vi "Main.vi"() -> ()   [LabVIEW 2021, in "Main.lvlib"]
uses:
  Main.lvlib
  Init/ReadInitCFG/TypeDef/CFG_Cluster.ctl
  TimeBasedProd/TimeTable/TypeDef/Time_Table.ctl
  TimeBasedProd/TimeTable/TypeDef/Time_Table_CTR.ctl
  TimeBasedProd/Digital_OP/TypeDef/Plant_OP_Map.ctl
  TimeBasedProd/Digital_OP/TypeDef/Plant_OP_Map_CTR.ctl
  ValveCTRL/TypeDef/CHs_List.ctl
  ValveCTRL/TypeDef/ChannelStatus.ctl
  ValveCTRL/TypeDef/Read_Write.ctl
  TimeBasedProd/TypeDef/Read_Write.ctl
  TimeBasedProd/TypeDef/TimeOutInfo.ctl
  ValveCTRL/TypeDef/Queue_Cluster.ctl
  ValveCTRL/TypeDef/States_Enum.ctl
  TimeBasedProd/TypeDef/UpdateTimeOutinfo.ctl
  Init/ReadInitCFG/TypeDef/Operation.ctl
  TimeBasedProd/TimeBasedProd.lvlib
  ValveCTRL/ValveCTRL.lvlib
  Temp_AS6200/Temp_AS6200.lvlib
panel:
  out "CHSt":T1
  in  "Plants_Digital_OP":T2 {"Channel No" items=["7"=7, "11"=11, "12"=12, "13"=13, "15"=15, "16"=16, "18"=18, "29"=29, "32"=32, "33"=33, "35"=35, "36"=36, "37"=37, "38"=38, "40"=40]}
  in  "Time Table":T5 {"Liter" min=0.0; "Set Time" format="%<%H:%M:%S>t"; "Duration[S]" min=0.0}
  in  "cmd":string
  in  "SendCMD":bool
  in  "CFG":T7 {"SystemResetTime" format="%<%H:%M:%S>t"}
  # "Valve -Open Valve -38 -10\nValve -Open Pump -38 -10\nValve -Wait Valve -38 -10\nValve -Close Pump -38 -10\nValve -Close Valve -38 -10"
  # "Event -[Init_IOs,ReadTimeTable,WrtTimeTable,ReadDigitalOP,WrtDigitalOP,CalcTimeOut,UpdateTimeOut,Stop] ;support multi\nTemp -[WrtTemp,Read,Stop] ;support multi\nValve -State[Open Valve,Open Pump,Wait Valve,Close Pump,Close Valve,Save State,StopLoop] -ChNo[7,11,12,13,15,16,18,29,32,33,35,36,37,38,40] - Duration\nStop -All\n         -Prod_All\n         -Prod_PC\n         -Prod_PI\n         -Event\n         -Temp\n         -Valve"
  # ">Stop the LabVIEW run-time:\nsudo systemctl stop labview.service\n>Start the LabVIEW run-time.\nsudo systemctl start labview.service"
  # "Watering Days"
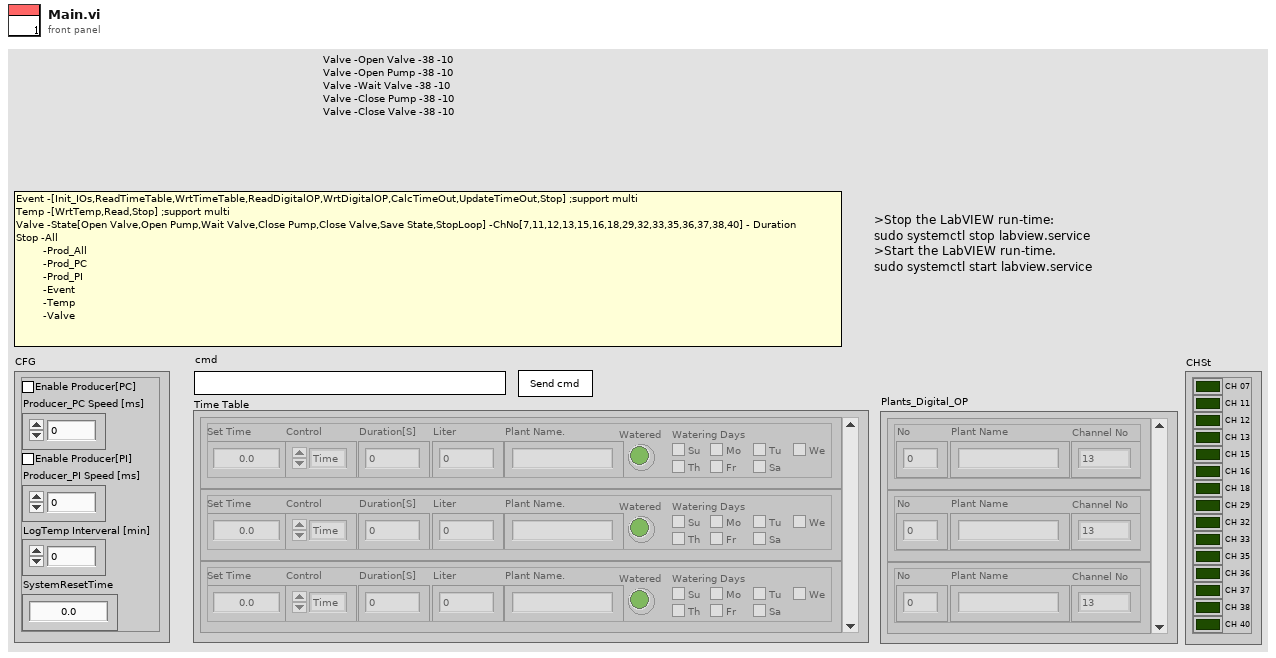
[diagram p1: front panel]
types:
  T1 = typedef "ValveCTRL.lvlib/ChannelStatus.ctl" = cluster{"CH 07":bool, "CH 11":bool, "CH 12":bool, "CH 13":bool, "CH 15":bool, "CH 16":bool, "CH 18":bool, "CH 29":bool, "CH 32":bool, "CH 33":bool, "CH 35":bool, "CH 36":bool, "CH 37":bool, "CH 38":bool, "CH 40":bool}
  T2 = typedef "TimeBasedProd.lvlib/Plant_OP_Map.ctl" = T3[]
  T3 = typedef "TimeBasedProd.lvlib/Plant_OP_Map_CTR.ctl" = cluster{"No":u8, "Plant Name":string, "Channel No":T4}
  T4 = typedef "ValveCTRL.lvlib/CHs_List.ctl" = u8
  T5 = typedef "TimeBasedProd.lvlib/Time_Table.ctl" = T6[]
  T6 = typedef "TimeBasedProd.lvlib/Time_Table_CTR.ctl" = cluster{"Set Time":dbl, "Control":enum16{"Time", "Flow"}, "Duration[S]":dbl, "Liter":dbl, "Plant Name.":string, "Watered":bool, "Su":bool, "Mo":bool, "Tu":bool, "We":bool, "Th":bool, "Fr":bool, "Sa":bool}
  T7 = typedef "Main.lvlib/CFG_Cluster.ctl" = cluster{"ProducerEn_PC":bool, "Producer_PC_ms":u32, "ProducerEn_PI":bool, "Producer_PI_ms":u32, "TempLogInterval":u32, "SystemResetTime":dbl}
  T8 = typedef "Main.lvlib/Operation.ctl" = enum16{"Write", "Read"}
  T9 = typedef "TimeBasedProd.lvlib/Read_Write.ctl" = cluster{"Time Table":T5, "Plants_Digital_OP":T2, "delta_ms_w_Index":T10, "TimeOutInfo":T13, "LoopName":string}
  T10 = typedef "TimeBasedProd.lvlib/TimeOutInfo.ctl" = cluster{"delta_ms":i32[], "Index":i32[], "RunArray":T11[]}
  T11 = typedef "ValveCTRL.lvlib/Queue_Cluster.ctl" = cluster{"State":T12, "Channel No":T4, "Duration[S]":dbl}
  T12 = typedef "ValveCTRL.lvlib/States_Enum.ctl" = enum16{"Open Pump", "Open Valve", "Wait Valve", "Close Pump", "Close Valve", "Save State", "StopLoop", "ValidCh"}
  T13 = typedef "TimeBasedProd.lvlib/UpdateTimeOutinfo.ctl" = cluster{"Timeout":i32, "ValveCTR":T11, "Index":i32}
  T14 = typedef "ValveCTRL.lvlib/Read_Write.ctl" = cluster{"CHSt":T1, "CH_Stat":bool, "ValidCh":T4[]}
  T15 = typedef "Main.lvlib/ReadOnly.ctl" = cluster{"Qref":cluster{"ValveCTR":refnum<queue>, "Error":refnum<queue>}, "UI_EN":bool, "UserEventREF":cluster{"TimeBasedProducer":cluster{"Reg":refnum<event-registration>, "Ref":refnum<user-event>}, "TimeBasedTempRead":cluster{"Reg":refnum<event-registration>, "Ref":refnum<user-event>}}, "UI_REF":variant, "Paths":cluster{"Log_Dir":path, "TempLog":path, "WateringLog":path, "Error":path, "Settings_Dir":path, "CFG.ini":path, "Plant_Digital_OP":path, "TimeTable":path, "Consol_Dir":path, "Input":path, "Output":path, "Timeout":path, "TimeoutTable":path, "Ch_Stat":path, "Temp":path}, "PI_REF":T16, "CFG":T7}
  T16 = typedef "LMH-LINX.lvlib/LINX Ref.ctl" = cluster{"IO":T17, "Interface":T18, "LINX Device Config":T19}
  T17 = typedef "LMH-LINX.lvlib/Platform.ctl" = enum16{"Remote", "Local"}
  T18 = typedef "LMH-LINX.lvlib/Interface.ctl" = enum16{"Serial", "TCP"}
  T19 = typedef "LMH-LINX.lvlib/Device.lvlib/LINX Device Config.ctl" = cluster{"Interface":T18, "COM Port":refnum<visa-resource-name>, "TCP Configuration":T20, "Device Family":u8, "Device ID":u8, "Device Name":string, "TCP Ref":refnum<k5>, "Channels":T21}
  T20 = typedef "LMH-LINX.lvlib/Device.lvlib/TCP Config.ctl" = cluster{"IP Address":string, "Port":u16}
  T21 = typedef "LMH-LINX.lvlib/Channels.ctl" = cluster{"DI":u8[], "DO":u8[], "AI":u8[], "AO":u8[], "PWM":u8[], "QE":u8[], "UART":u8[], "I2C 2":u8[], "SPI":u8[], "CAN":u8[], "Servo":u8[], "AI Ref (V)":dbl, "AI Resolution (Bits)":u8, "AO Ref (V)":dbl, "AO Resolution (Bits)":u8}
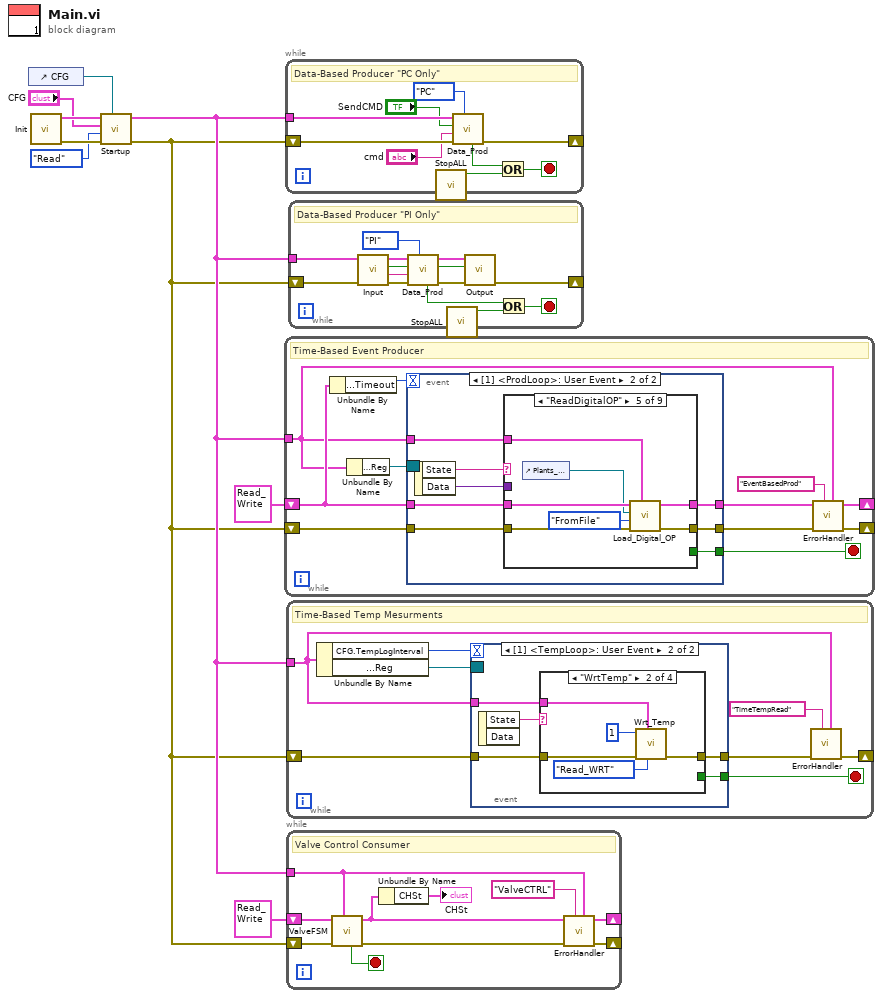
[diagram p0: block diagram]
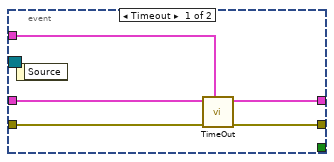
[diagram p2: hidden frame]
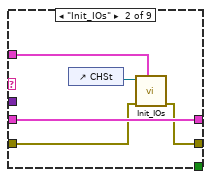
[diagram p4: hidden frame]
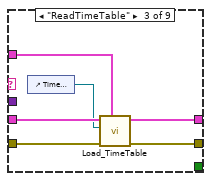
[diagram p5: hidden frame]
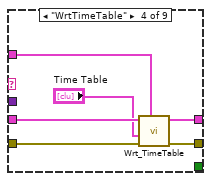
[diagram p6: hidden frame]
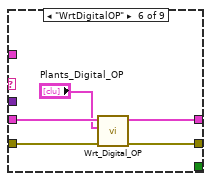
[diagram p7: hidden frame]
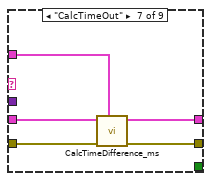
[diagram p8: hidden frame]
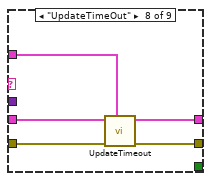
[diagram p9: hidden frame]
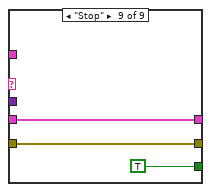
[diagram p10: hidden frame]
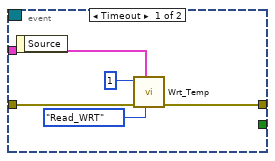
[diagram p11: hidden frame]
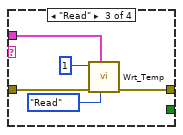
[diagram p13: hidden frame]
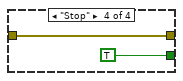
[diagram p14: hidden frame]
diagram:
  n1 = control-ref of="CFG"() -> (w4:refnum<vi>)
  n2 = call "Init.vi"() -> ("error out"=w8:errorcluster, "ReadOnly"=w7:T15)  [unwired: 10 in]
  n3 = call "Startup.vi"(7:"CFG"=w4, "error in"=w8, "Operation"=Operation."Read", 10:"CFG"="CFG", "ReadOnlyIn"=w7) -> ("error out"=w1:errorcluster, "ReadOnlyOut"=w3:T15)  [unwired: 5 in]
  n4 = while {
    shift-right: [w13] -> _
    shift-left: w1 -> [w18]
    tunnel: w3 -> [w12]
    shift-right: [w10] -> _
    shift-left: T9 {"Time Table"=[], "Plants_Digital_OP"=[], "delta_ms_w_Index"={"delta_ms"=[], "Index"=[], "RunArray"=[]}, "TimeOutInfo"={"Timeout"=0, "ValveCTR"={"State"=enum."Open Valve", "Channel No"=0, "Duration[S]"=0.0}, "Index"=0}, "LoopName"="TimeBasedEvent"} ("Read_Write") -> [w16]
    stop <- w17 stop-if-true
    # "Time-Based Event Producer"
    n5 = Unbundle By Name(w16) -> ("TimeOutInfo.Timeout"=w15:i32)
    n6 = Unbundle By Name(w12) -> ("UserEventREF.TimeBasedProducer.Reg"=w19:refnum<event-registration>)
    n7 = event shown="[1] <ProdLoop>: User Event" {
      selector: w19 -> [_ _]
      dyn-events: _ -> [_ _]
      timeout: w15 -> [_ _]
      tunnel: w18 -> [w24 w30]
      tunnel: [w23 w29] -> w14
      tunnel: [_ w28] -> w17
      tunnel: w12 -> [w20 w27]
      tunnel: w16 -> [w22 w26]
      tunnel: [w21 w25] -> w10
      event Timeout {
        n8 = event-data() -> ()  [unwired: 1 in, 1 out]
        n9 = call "TimeOut.vi"("ReadOnlyIn"=w20, "error in"=w24, "Read_WriteIIN"=w22) -> ("error out"=w23:errorcluster, "Read_WriteIIOUT"=w21:T9)  [unwired: 7 in]
      }
      event User Event {
        n10 = event-data() -> ("State"=w32:string, "Data"=w31:variant)  [unwired: 1 in]
        n11 = case shown="\"ReadDigitalOP\"" w32 {
          tunnel: w31 -> [_ _ _ _ _ _ _ _ _]
          tunnel: w30 -> [w34 w38 w45 w51 w58 w63 w68 w72 w76]
          tunnel: [w34 w37 w44 w50 w57 w62 w67 w71 w76] -> w29
          tunnel: [_ _ _ _ _ _ _ _ TRUE] -> w28
          tunnel: w27 -> [_ w36 w43 w49 w54 _ w64 w69 _]
          tunnel: w26 -> [w33 w39 w42 w48 w56 w61 w66 w73 w74]
          tunnel: [w33 w39 w41 w47 w55 w60 w65 w70 w74] -> w25
          frame Default {
          }
          frame "Init_IOs" {
            n12 = control-ref of="CHSt"() -> (w35:refnum<vi>)
            n13 = call "Init_IOs.vi"("ReadOnlyIn"=w36, "error in"=w38, "CHSt"=w35) -> ("error out"=w37:errorcluster)  [unwired: 8 in]
          }
          frame "ReadTimeTable" {
            n14 = control-ref of="Time Table"() -> (w40:refnum<vi>)
            n15 = call "Load_TimeTable.vi"("ReadOnly"=w43, "Error In"=w45, "Time Table"=w40, "Read_WriteIN"=w42) -> ("Error Out"=w44:errorcluster, "Read_WriteIOUT"=w41:T9)  [unwired: 6 in]
          }
          frame "WrtTimeTable" {
            n16 = call "Wrt_TimeTable.vi"("ReadOnlyIn"=w49, "Error In"=w51, "Time Table In"="Time Table", "Read_WriteIN"=w48) -> ("Error Out"=w50:errorcluster, "Read_WriteOUT"=w47:T9)  [unwired: 6 in]
          }
          frame "ReadDigitalOP" {
            n17 = control-ref of="Plants_Digital_OP"() -> (w53:refnum<vi>)
            n18 = call "Load_Digital_OP.vi"("ReadOnlyIn"=w54, "Error In"=w58, "Oper"=enum16{"FromFile", "FromMem"}."FromFile", "Plants_Digital_OP"=w53, "Read_WriteIN"=w56) -> ("Error Out"=w57:errorcluster, "Read_WriteIOUT"=w55:T9)  [unwired: 4 in, 1 out]
          }
          frame "WrtDigitalOP" {
            n19 = call "Wrt_Digital_OP.vi"("Error In"=w63, "Plants_Digital_OP"="Plants_Digital_OP", "Read_WriteIN"=w61) -> ("Error Out"=w62:errorcluster, "Read_WriteIOUT"=w60:T9)  [unwired: 7 in]
          }
          frame "CalcTimeOut" {
            n20 = call "CalcTimeDifference_ms.vi"("ReadOnlyIm"=w64, "Error In"=w68, "Read_WriteIN"=w66) -> ("Error Out"=w67:errorcluster, "Read_WriteOUT"=w65:T9)  [unwired: 6 in, 1 out]
          }
          frame "UpdateTimeOut" {
            n21 = call "UpdateTimeout.vi"("ReadOnlyIn"=w69, "Error In"=w72, "Read_WriteIN"=w73) -> ("Error Out"=w71:errorcluster, "Read_WriteOUT"=w70:T9)  [unwired: 7 in]
          }
          frame "Stop" {
          }
        }
      }
    }
    n22 = call "ErrorHandler.vi"("ReadOnlyIn"=w12, "LoopName"="EventBasedProd", "error in"=w14) -> ("error out"=w13:errorcluster)  [unwired: 8 in]
  }
  n23 = while {
    tunnel: w3 -> [w84]
    shift-right: [w82] -> _
    shift-left: w1 -> [w85]
    stop <- w77 stop-if-true
    # "Data-Based Producer \"PC Only\""
    n24 = call "StopALL.vi"() -> ("StopOUT"=w78:bool)  [unwired: 11 in]
    n25 = call "Data_Prod.vi"("ProdType"=enum16{"PC", "PI"}."PC", "error in"=w85, "cmd"="cmd", "SendCMD"="SendCMD", "ReadOnlyIn"=w84) -> ("error out"=w82:errorcluster, "Stop"=w79:bool)  [unwired: 3 in, 2 out]
    n26 = Or(x=w79, y=w78) -> (x .or. y?=w77:bool)
  }
  n27 = while {
    shift-right: [w88] -> _
    shift-left: w1 -> [w93]
    tunnel: w3 -> [w86]
    stop <- w91 stop-if-true
    # "Time-Based Temp Mesurments"
    n28 = Unbundle By Name(w86) -> ("CFG.TempLogInterval"=w90:u32, "UserEventREF.TimeBasedTempRead.Reg"=w92:refnum<event-registration>)
    n29 = event shown="[1] <TempLoop>: User Event" {
      selector: w92 -> [_ _]
      dyn-events: _ -> [_ _]
      timeout: w90 -> [_ _]
      tunnel: w93 -> [w98 w103]
      tunnel: [w97 w101] -> w89
      tunnel: [_ w100] -> w91
      tunnel: w86 -> [w94 w99]
      event Timeout {
        n30 = event-data() -> ()  [unwired: 1 in, 1 out]
        n31 = call "Wrt_Temp.vi"("Oper"=enum16{"Read", "Read_WRT"}."Read_WRT", "ReadOnlyIn"=w94, "error in"=w98, "I2C Channel"=u8 1) -> ("error out"=w97:errorcluster)  [unwired: 6 in, 1 out]
      }
      event User Event {
        n32 = event-data() -> ("State"=w102:string)  [unwired: 1 in, 1 out]
        n33 = case shown="\"WrtTemp\"" w102 {
          tunnel: w103 -> [w104 w109 w114 w115]
          tunnel: [w104 w108 w113 w115] -> w101
          tunnel: [_ _ _ TRUE] -> w100
          tunnel: w99 -> [_ w105 w110 _]
          frame Default {
          }
          frame "WrtTemp" {
            n34 = call "Wrt_Temp.vi"("Oper"=enum16{"Read", "Read_WRT"}."Read_WRT", "ReadOnlyIn"=w105, "error in"=w109, "I2C Channel"=u8 1) -> ("error out"=w108:errorcluster)  [unwired: 6 in, 1 out]
          }
          frame "Read" {
            n35 = call "Wrt_Temp.vi"("Oper"=enum16{"Read", "Read_WRT"}."Read", "ReadOnlyIn"=w110, "error in"=w114, "I2C Channel"=u8 1) -> ("error out"=w113:errorcluster)  [unwired: 6 in, 1 out]
          }
          frame "Stop" {
          }
        }
      }
    }
    n36 = call "ErrorHandler.vi"("ReadOnlyIn"=w86, "LoopName"="TimeTempRead", "error in"=w89) -> ("error out"=w88:errorcluster)  [unwired: 8 in]
  }
  n37 = while {
    shift-right: [w121] -> _
    shift-left: w1 -> [w125]
    tunnel: w3 -> [w120]
    shift-right: [w118] -> _
    shift-left: T14 {"CHSt"={"CH 07"=FALSE, "CH 11"=FALSE, "CH 12"=FALSE, "CH 13"=FALSE, "CH 15"=FALSE, "CH 16"=FALSE, "CH 18"=FALSE, "CH 29"=FALSE, "CH 32"=FALSE, "CH 33"=FALSE, "CH 35"=FALSE, "CH 36"=FALSE, "CH 37"=FALSE, "CH 38"=FALSE, "CH 40"=FALSE}, "CH_Stat"=FALSE, "ValidCh"=[]} ("Read_Write_Valv") -> [w124]
    stop <- w123 stop-if-true
    # "Valve Control Consumer"
    n38 = call "ValveFSM.vi"("ReadOnlyIn"=w120, "error in"=w125, "Read_Write_Valv_IN"=w124) -> ("error out"=w122:errorcluster, "Read_Write_Valv_OUT"=w118:T14, "Stop"=w123:bool)  [unwired: 6 in]
    n39 = Unbundle By Name(w118) -> ("CHSt"=→"CHSt":T1)
    n40 = call "ErrorHandler.vi"("ReadOnlyIn"=w120, "LoopName"="ValveCTRL", "error in"=w122) -> ("error out"=w121:errorcluster)  [unwired: 8 in]
  }
  n41 = while {
    tunnel: w3 -> [w137]
    shift-right: [w132] -> _
    shift-left: w1 -> [w139]
    stop <- w127 stop-if-true
    # "Data-Based Producer \"PI Only\""
    n42 = call "Input.vi"("error in (no error)"=w139, "ReadOnlyIn"=w137) -> ("error out"=w138:errorcluster, "cmd"=w134:string, "SendCMD"=w135:bool, "ReadOnlyIOut"=w136:T15)  [unwired: 6 in]
    n43 = call "Data_Prod.vi"("ProdType"=enum16{"PC", "PI"}."PI", "error in"=w138, "cmd"=w134, "SendCMD"=w135, "ReadOnlyIn"=w136) -> ("error out"=w133:errorcluster, "SendCMD"=w126:bool, "ReadOnlyOut"=w131:T15, "Stop"=w128:bool)  [unwired: 3 in]
    n44 = call "StopALL.vi"() -> ("StopOUT"=w129:bool)  [unwired: 11 in]
    n45 = call "Output.vi"("error in (no error)"=w133, "SendCMD"=w126, "ReadOnlyIIn"=w131) -> ("error out"=w132:errorcluster)  [unwired: 8 in]
    n46 = Or(x=w128, y=w129) -> (x .or. y?=w127:bool)
  }
